vi "AppendViName.vi"(8 "error in (no error)":errorcluster, 10 "VI Refnum":refnum<vi>, 11 "MockListImp in":refnum<class "ListImp_RefSpy.lvclass">) -> (0 "error out":errorcluster, 3 "MockListImp out":refnum<class "ListImp_RefSpy.lvclass">)   [LabVIEW 2013, in "ListImp_RefSpy.lvclass"]
uses:
  ListImp_RefSpy.lvclass
  RefnumGlobal.vi
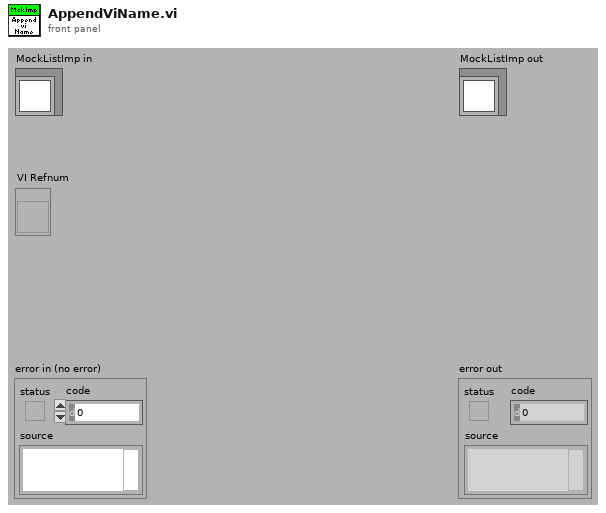
[diagram p1: front panel]
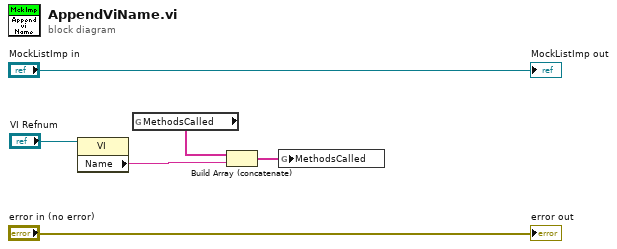
[diagram p0: block diagram]
diagram:
  n1 = property class="VI"(reference="VI Refnum") -> ("Name"=w4:string)  [unwired: 1 in, 2 out]
  n2 = global read "RefnumGlobal.vi" "MethodsCalled"() -> (w1:string[])
  n3 = Build Array (concatenate)(w1, w4) -> (w2:string[])
  n4 = global write "RefnumGlobal.vi" "MethodsCalled"(w2) -> ()
  "error out" <- "error in (no error)"
  "MockListImp out" <- "MockListImp in"
